vi "Select image acquisition mode.vi"(8 "error in (no error)":errorcluster, 11 "Autofocus in":refnum<class "Autofocus.lvclass">) -> (0 "error out":errorcluster, 3 "Autofocus out":refnum<class "Autofocus.lvclass">)   [LabVIEW 2012, in "Autofocus.lvclass"]
uses:
  Autofocus.lvclass
  Autofocus.lvclass/Autofocus.ctl
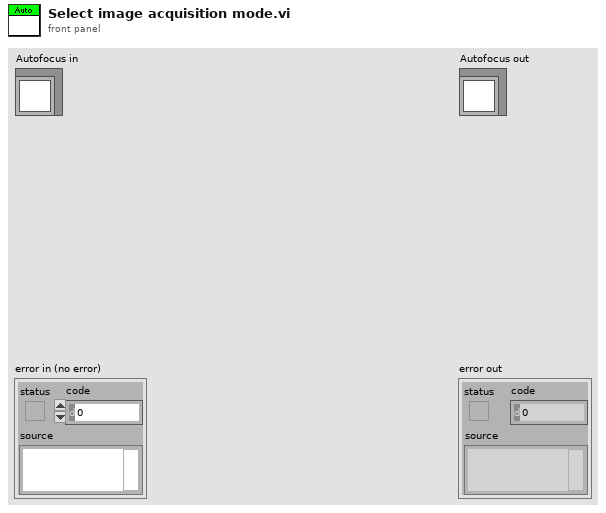
[diagram p1: front panel]
types:
  T1 = typedef "Autofocus.lvclass/image acquisition mode.ctl" = enum16{"Focus Stack", "Single Frame"}
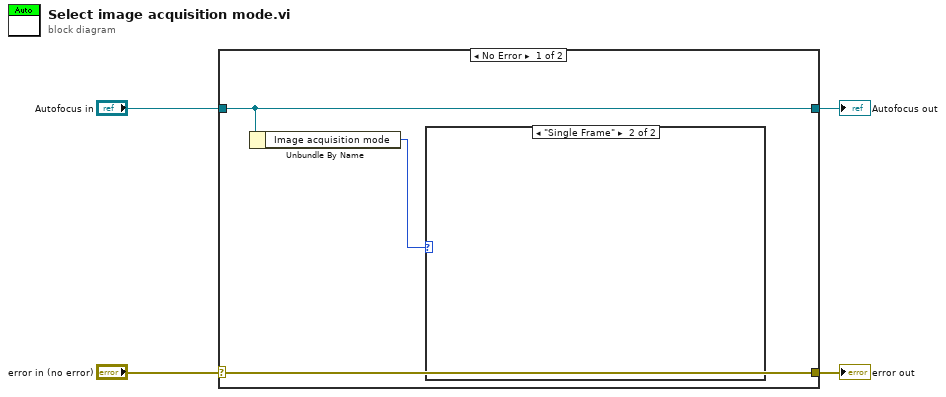
[diagram p0: block diagram]
diagram:
  n1 = case shown="No Error" "error in (no error)" {
    selector: "error in (no error)" -> [w7 w9]
    tunnel: [w7 w9] -> w3
    tunnel: [w6 w8] -> w1
    tunnel: "Autofocus in" -> [w6 w8]
    frame No Error {
      n2 = Unbundle By Name(w6) -> ("Image acquisition mode"=w5:T1)
      n3 = case shown="\"Single Frame\"" w5 {
        frame "Focus Stack", Default {
        }
        frame "Single Frame" {
        }
      }
    }
    frame Error {
    }
  }
  "error out" <- w3
  "Autofocus out" <- w1
